vi "4.7.vi"() -> ()   [LabVIEW 2017]
panel:
  out "随机数":dbl
  out "次数":dbl
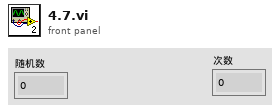
[diagram p1: front panel]
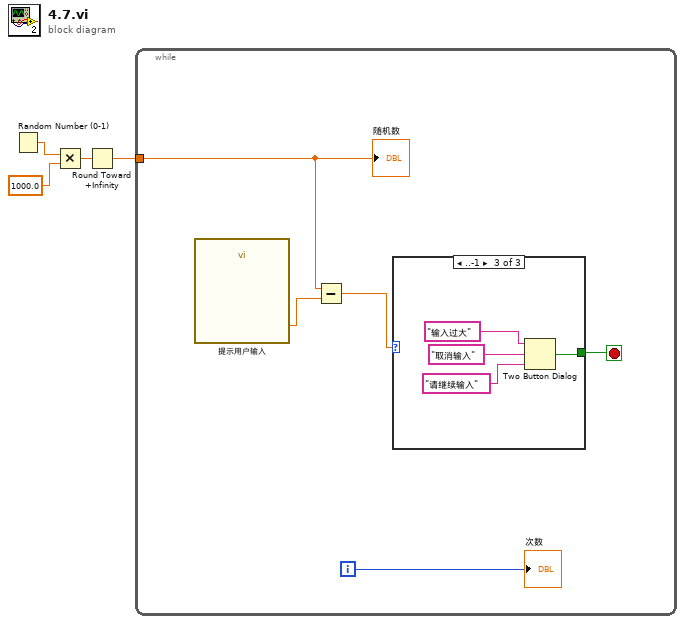
[diagram p0: block diagram]
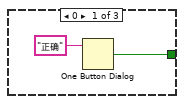
[diagram p2: hidden frame]
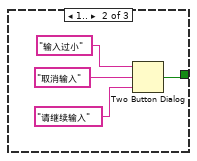
[diagram p3: hidden frame]
diagram:
  n1 = Random Number (0-1)() -> (number: 0 to 1=w4:dbl)
  n2 = Multiply(x=w4, y=1000.0) -> (x*y=w3:dbl)
  n3 = Round Toward +Infinity(x=w3) -> (ceil(x): smallest int >= x=w1:dbl)
  n4 = while {
    tunnel: w1 -> [w5]
    i -> [w9]
    stop <- w8 stop-if-true
    n5 = call "提示用户输入"() -> ("请输入1-1000"=w6:dbl)  [unwired: 17 in, 2 out]
    n6 = Subtract(x=w5, y=w6) -> (x-y=w7:dbl)
    n7 = case shown="..-1" w7 {
      tunnel: [w10 w12 w16] -> w8
      frame 0 {
        n8 = One Button Dialog(message="正确") -> (true=w10:bool)  [unwired: 1 in]
      }
      frame 1.. {
        n9 = Two Button Dialog(message="输入过小", 1:"请继续输入", 2:"取消输入") -> (T button?=w12:bool)
      }
      frame ..-1 {
        n10 = Two Button Dialog(message="输入过大", 1:"请继续输入", 2:"取消输入") -> (T button?=w16:bool)
      }
    }
    "次数" <- w9
    "随机数" <- w5
  }
